vi "Quit.vi"(8 "error in (no error)":errorcluster, 11 "tWorkerTCPConnection in":refnum<class "tWorkerCommandRunner.lvclass">) -> (0 "error out":errorcluster, 3 "tWorkerTCPConnection out":refnum<class "tWorkerCommandRunner.lvclass">)   [LabVIEW 2012]
uses:
  BSON/tBSONDocument/tBSONDocument.lvclass
  BSON/tBSONDocument/addStringElement.vi
  tWorkerCommandRunner.lvclass
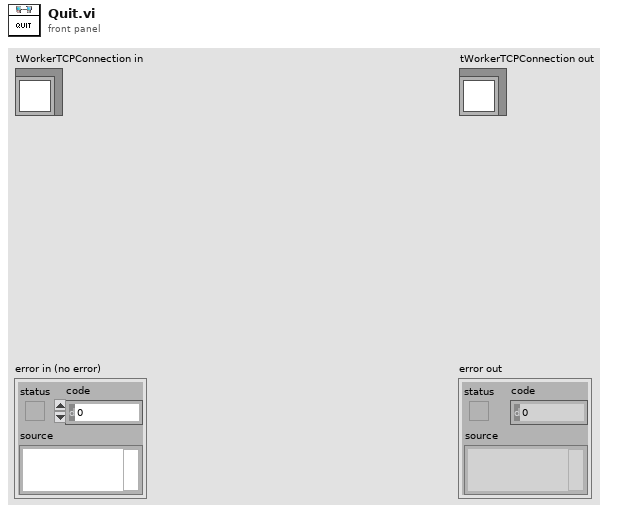
[diagram p1: front panel]
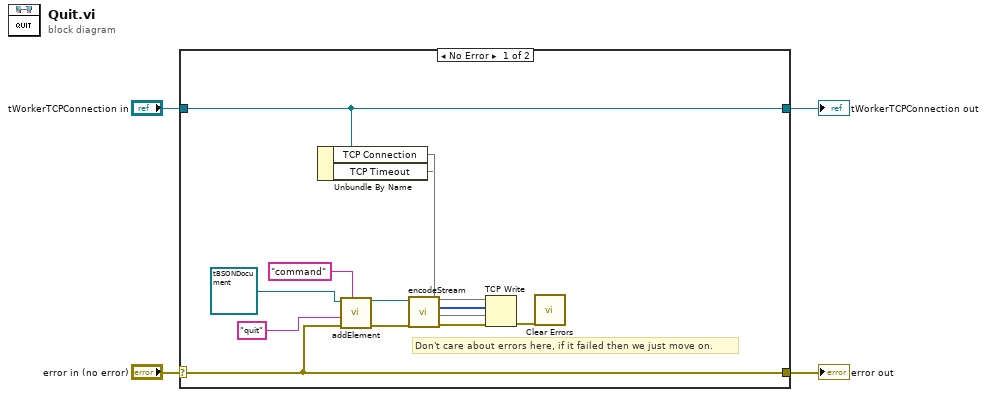
[diagram p0: block diagram]
diagram:
  n1 = case shown="No Error" "error in (no error)" {
    selector: "error in (no error)" -> [w6 w18]
    tunnel: [w6 w18] -> w3
    tunnel: [w9 w17] -> w1
    tunnel: "tWorkerTCPConnection in" -> [w9 w17]
    frame No Error {
      # "Don't care about errors here, if it failed then we just move on."
      n2 = Unbundle By Name(w9) -> ("TCP Connection"=w8, "TCP Timeout"=w7)
      n3 = call-poly "addElement.vi"("Name"="command", "error in (no error)"=w6, "Value"="quit", "tBSONDocument in"=refnum<class "tBSONDocument.lvclass"> refnum ("BSON.lvlib:tBSONDocument.lvclass")) -> ("error out"=w13:errorcluster, "tBSONDocument out"=w12:refnum<class "tBSONDocument.lvclass">)  [unwired: 6 in]
      n4 = call "encodeStream.vi"("error in (no error)"=w13, "tBSONDocument in"=w12) -> ("error out"=w11:errorcluster, "Byte Data"=w10:u8[])  [unwired: 7 in, 1 out]
      n5 = TCP Write(connection ID=w8, data in=w10, error in (no error)=w11, 9:w7) -> (error out=w5:errorcluster)  [unwired: 2 out]
      n6 = call <vilib>:"Clear Errors.vi"("error in (no error)"=w5) -> ()  [unwired: 6 in, 1 out]
    }
    frame Error {
    }
  }
  "error out" <- w3
  "tWorkerTCPConnection out" <- w1
